vi "Turret_Set.vi"   [LabVIEW 2019]
uses:
  Turret_Globals.vi
types:
  T1 = enum16{"Manual_PercentVoltage", "Manual_SpeedControl", "Auto_Targeting", "Position"}
  T2 = typedef "Turret_Cluster.ctl" = cluster{"Control_State":enum16{"Manual_PercentVoltage", "Manual_SpeedControl", "Auto_Targeting", "Position"}, "Spin_Power":dbl, "Flywheel_Power":dbl, "Going_To_Position":bool}
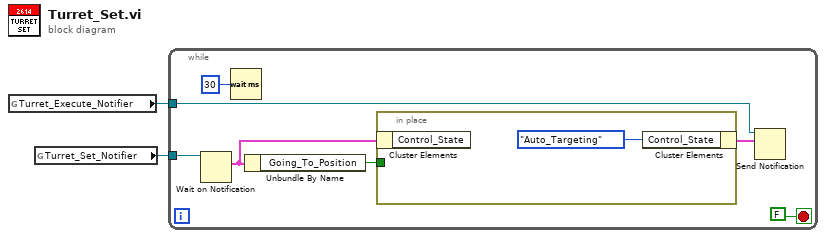
[diagram p0: block diagram]
diagram:
  n1 = global read "Turret_Globals.vi" "Turret_Execute_Notifier"() -> (w1:refnum<notifier>)
  n2 = global read "Turret_Globals.vi" "Turret_Set_Notifier"() -> (w2:refnum<notifier>)
  n3 = while {
    tunnel: w2 -> [w7]
    tunnel: w1 -> [w5]
    stop <- FALSE stop-if-true
    n4 = Wait on Notification(notifier=w7) -> (notification=w4:T2)  [unwired: 3 in, 3 out]
    n5 = Wait (ms)(milliseconds to wait=u32 30) -> ()  [unwired: 1 out]
    n6 = Unbundle By Name(w4) -> ("Going_To_Position"=w3:bool)
    n7 = in-place {
      in-place-border: w3 -> [_]
      n8 = in-place-cluster #1(w4) -> ()  [unwired: 1 out]
      n9 = in-place-cluster #1("Control_State"=T1."Auto_Targeting") -> (w6:T2)
    }
    n10 = Send Notification(notification=w6, notifier=w5) -> ()  [unwired: 1 in, 2 out]
  }
